vi "Send To Creator.vi"(4 "Is Priority":bool, 7 "Actor in":refnum<class "Actor.lvclass">) -> (0 "Error out":errorcluster)   [LabVIEW 2025, in "jettl.lvlib" / "Destroy Msg.lvlib"]
uses:
  Destroy Msg.lvlib
  Actor/Actor/Actor.lvclass
  Destroy Msg/Destroy Msg.lvclass
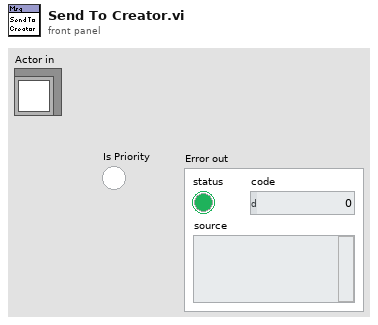
[diagram p1: front panel]
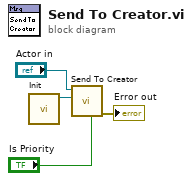
[diagram p0: block diagram]
diagram:
  n1 = call "Init.vi"() -> ("Destroy Msg out"=w1:refnum<class "Destroy Msg.lvclass">)  [unwired: 11 in]
  n2 = call-dynamic "Send To Creator.vi"("Is Priority"="Is Priority", "Msg"=w1, "Actor in"="Actor in") -> ("Error out"=→"Error out":errorcluster)  [unwired: 8 in]
